vi "CSGaussmeter.openGUI.vi"(11 "error in":errorcluster) -> (15 "error out":errorcluster)   [LabVIEW 2014, in "CSGaussmeter.lvlib"]
uses:
  CSGaussmeter.lvlib
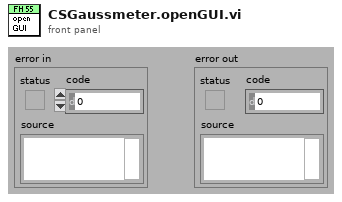
[diagram p1: front panel]
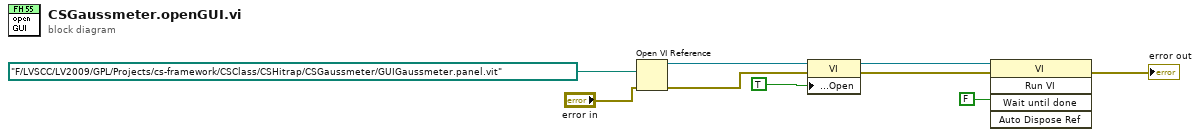
[diagram p0: block diagram]
diagram:
  n1 = Open VI Reference(vi path=path "F:/LVSCC/LV2009/GPL/Projects/cs-framework/CSClass/CSHitrap/CSGaussmeter/GUIGaussmeter.panel.vit", error in (no error)="error in") -> (vi reference=w7:refnum<vi>, error out=w6:errorcluster)  [unwired: 4 in]
  n2 = property class="VI"(reference=w7, error in=w6, "Front Panel.Open"=TRUE) -> (reference out=w4:refnum<vi>, error out=w3:errorcluster)
  n3 = invoke class="VI" method="Run VI"(reference=w4, error in=w3, "Wait until done"=FALSE ("Wait Until Done")) -> (error out=→"error out":errorcluster)  [unwired: 2 in, 4 out]
